vi "slider driver -- real.vi"(0 "slider in":refnum<vi>, 1 "slider action":T1, 9 "slider from":refnum<vi>, 11 "value IN":dbl=5700.934579439253, 12 "default":dbl=5700.934579439253) -> (4 "slider out":refnum<vi>, 6 "max":dbl, 8 "rel OUT":dbl, 10 "min":dbl, 15 "value OUT":dbl=5700.934579439253)   [LabVIEW 2018]
uses:
  slider action.ctl
  Q - not nan -- real.vi
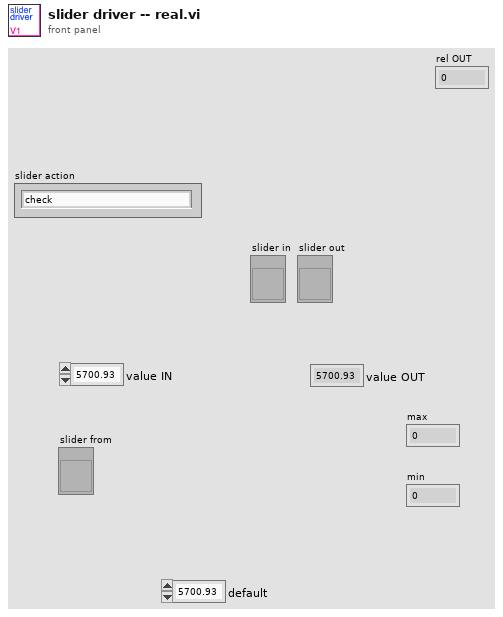
[diagram p1: front panel]
types:
  T1 = typedef "slider action.ctl" = enum16{"check", "copy range", "set from value", "set from ratio", "set from slider", "read using other slider", "set lower limit", "set upper limit", "set lower from slider", "set upper from slider"}
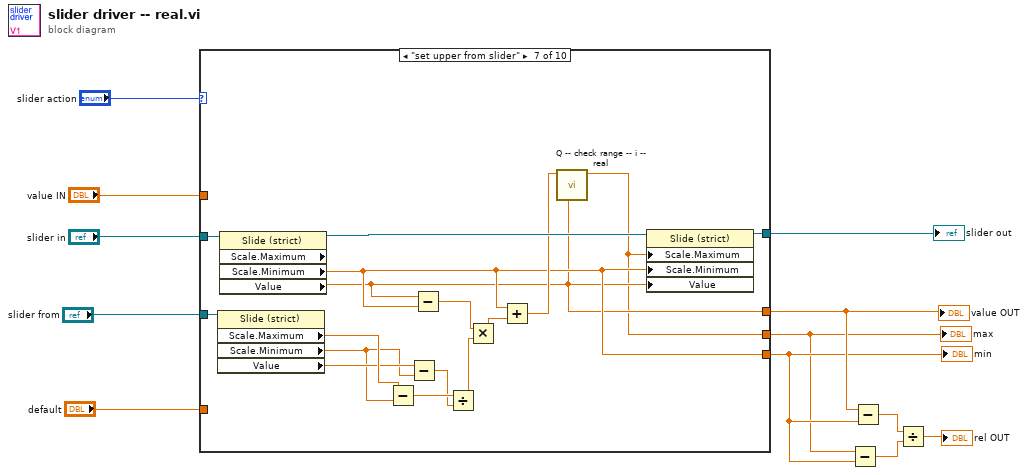
[diagram p0: block diagram]
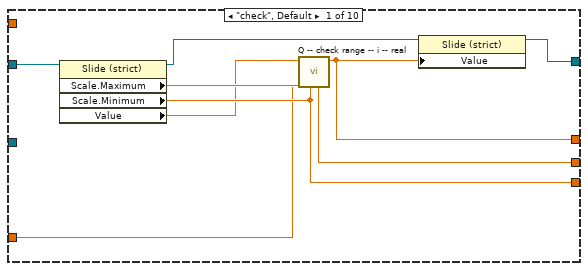
[diagram p2: hidden frame]
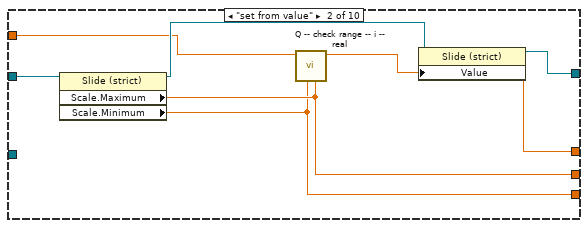
[diagram p3: hidden frame]
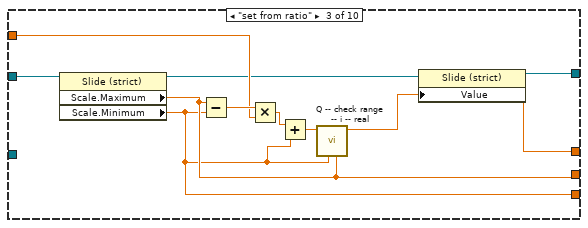
[diagram p4: hidden frame]
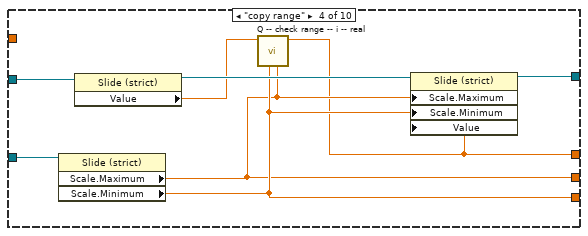
[diagram p5: hidden frame]
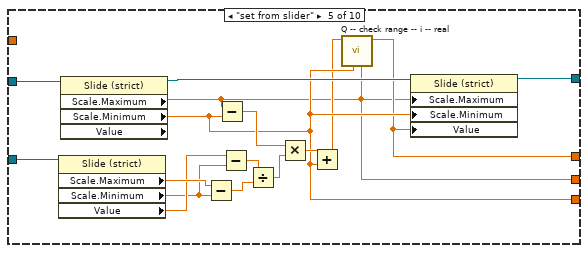
[diagram p6: hidden frame]
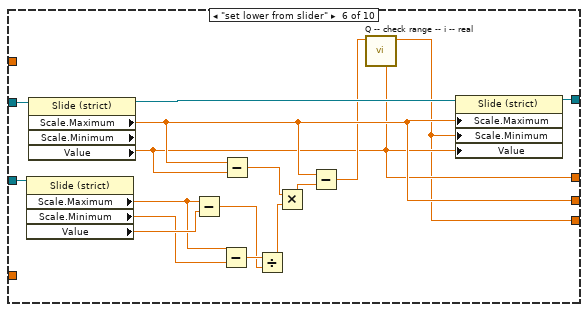
[diagram p7: hidden frame]
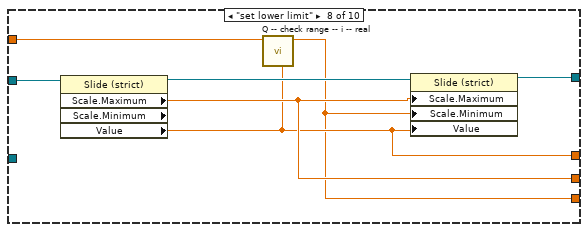
[diagram p8: hidden frame]
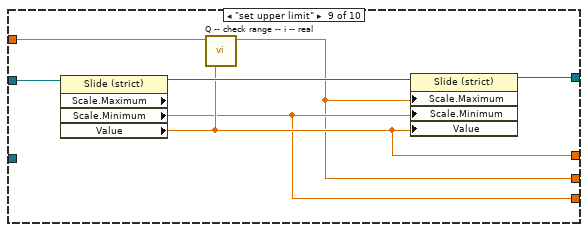
[diagram p9: hidden frame]
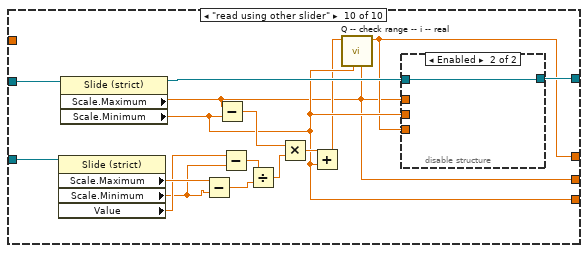
[diagram p10: hidden frame]
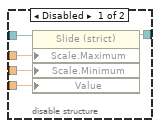
[diagram p11: hidden frame]
diagram:
  n1 = case shown="\"set upper from slider\"" "slider action" {
    tunnel: "slider in" -> [w20 w27 w37 w43 w59 w75 w91 w99 w106 w121]
    tunnel: [w19 w26 w36 w38 w47 w63 w79 w95 w103 w109] -> w6
    tunnel: [w17 w24 w35 w44 w60 w76 w92 w100 w107 w122] -> w2
    tunnel: "slider from" -> [_ _ _ w45 w61 w77 w93 _ _ w123]
    tunnel: [w15 w22 w30 w40 w49 w62 w80 w94 w102 w111] -> w5
    tunnel: [w16 w23 w34 w39 w46 w66 w78 w97 w101 w108] -> w4
    tunnel: "value IN" -> [_ w21 w32 _ _ _ _ w98 w105 _]
    tunnel: "default" -> [w14 _ _ _ _ _ _ _ _ _]
    frame "check", Default {
      n2 = property class="Slide (strict)"(reference=w20) -> (reference out=w18:refnum<vi>, "Scale.Maximum"=w16:dbl, "Scale.Minimum"=w15:dbl, "Value"=w13:dbl)  [unwired: 1 in, 1 out]
      n3 = call "Q -- check range -- i -- real.vi"("upper"=w16, "lower"=w15, "default"=w14, "number"=w13) -> ("number in range"=w19:dbl)  [unwired: 5 in, 2 out]
      n4 = property class="Slide (strict)"(reference=w18, "Value"=w19) -> (reference out=w17:refnum<vi>)  [unwired: 1 in, 1 out]
    }
    frame "set from value" {
      n5 = property class="Slide (strict)"(reference=w27) -> (reference out=w25:refnum<vi>, "Scale.Maximum"=w23:dbl, "Scale.Minimum"=w22:dbl)  [unwired: 1 in, 1 out]
      n6 = call "Q -- check range -- i -- real.vi"("upper"=w23, "lower"=w22, "number"=w21) -> ("number in range"=w26:dbl)  [unwired: 6 in, 2 out]
      n7 = property class="Slide (strict)"(reference=w25, "Value"=w26) -> (reference out=w24:refnum<vi>)  [unwired: 1 in, 1 out]
    }
    frame "set from ratio" {
      n8 = property class="Slide (strict)"(reference=w37) -> (reference out=w31:refnum<vi>, "Scale.Maximum"=w34:dbl, "Scale.Minimum"=w30:dbl)  [unwired: 1 in, 1 out]
      n9 = Subtract(x=w34, y=w30) -> (x-y=w33:dbl)
      n10 = Multiply(x=w33, y=w32) -> (x*y=w29:dbl)
      n11 = Add(x=w29, y=w30) -> (x+y=w28:dbl)
      n12 = call "Q -- check range -- i -- real.vi"("upper"=w34, "lower"=w30, "number"=w28) -> ("number in range"=w36:dbl)  [unwired: 6 in, 2 out]
      n13 = property class="Slide (strict)"(reference=w31, "Value"=w36) -> (reference out=w35:refnum<vi>)  [unwired: 1 in, 1 out]
    }
    frame "copy range" {
      n14 = property class="Slide (strict)"(reference=w45) -> ("Scale.Maximum"=w39:dbl, "Scale.Minimum"=w40:dbl)  [unwired: 1 in, 2 out]
      n15 = property class="Slide (strict)"(reference=w43) -> (reference out=w42:refnum<vi>, "Value"=w41:dbl)  [unwired: 1 in, 1 out]
      n16 = call "Q -- check range -- i -- real.vi"("upper"=w39, "lower"=w40, "number"=w41) -> ("number in range"=w38:dbl)  [unwired: 6 in, 2 out]
      n17 = property class="Slide (strict)"(reference=w42, "Scale.Maximum"=w39, "Scale.Minimum"=w40, "Value"=w38) -> (reference out=w44:refnum<vi>)  [unwired: 1 in, 1 out]
    }
    frame "set from slider" {
      n18 = property class="Slide (strict)"(reference=w61) -> ("Scale.Maximum"=w57:dbl, "Scale.Minimum"=w55:dbl, "Value"=w56:dbl)  [unwired: 1 in, 2 out]
      n19 = property class="Slide (strict)" props=["Scale", "Maximum", "Scale", "Minimum", "Value"](reference=w59) -> (reference out=w58:refnum<vi>, "Scale.Maximum"=w46:dbl, "Scale.Minimum"=w49:dbl)  [unwired: 1 in, 2 out]
      n20 = Subtract(x=w57, y=w55) -> (x-y=w53:dbl)
      n21 = Subtract(x=w46, y=w49) -> (x-y=w51:dbl)
      n22 = Subtract(x=w56, y=w55) -> (x-y=w54:dbl)
      n23 = Divide(x=w54, y=w53) -> (x/y=w52:dbl)
      n24 = Multiply(x=w51, y=w52) -> (x*y=w50:dbl)
      n25 = Add(x=w50, y=w49) -> (x+y=w48:dbl)
      n26 = call "Q -- check range -- i -- real.vi"("upper"=w46, "lower"=w49, "number"=w48) -> ("number in range"=w47:dbl)  [unwired: 6 in, 2 out]
      n27 = property class="Slide (strict)"(reference=w58, "Scale.Maximum"=w46, "Scale.Minimum"=w49, "Value"=w47) -> (reference out=w60:refnum<vi>)  [unwired: 1 in, 1 out]
    }
    frame "set lower from slider" {
      n28 = property class="Slide (strict)"(reference=w77) -> ("Scale.Maximum"=w71:dbl, "Scale.Minimum"=w70:dbl, "Value"=w72:dbl)  [unwired: 1 in, 2 out]
      n29 = property class="Slide (strict)" props=["Scale", "Maximum", "Scale", "Minimum", "Value"](reference=w75) -> (reference out=w74:refnum<vi>, "Scale.Maximum"=w66:dbl, "Value"=w63:dbl)  [unwired: 1 in, 2 out]
      n30 = Subtract(x=w71, y=w72) -> (x-y=w69:dbl)
      n31 = Subtract(x=w71, y=w70) -> (x-y=w73:dbl)
      n32 = Subtract(x=w66, y=w63) -> (x-y=w68:dbl)
      n33 = Divide(x=w73, y=w69) -> (x/y=w67:dbl)
      n34 = Multiply(x=w68, y=w67) -> (x*y=w65:dbl)
      n35 = Subtract(x=w66, y=w65) -> (x-y=w64:dbl)
      n36 = call "Q -- check range -- i -- real.vi"("upper"=w63, "number"=w64) -> ("number in range"=w62:dbl)  [unwired: 7 in, 2 out]
      n37 = property class="Slide (strict)"(reference=w74, "Scale.Maximum"=w66, "Scale.Minimum"=w62, "Value"=w63) -> (reference out=w76:refnum<vi>)  [unwired: 1 in, 1 out]
    }
    frame "set upper from slider" {
      n38 = property class="Slide (strict)"(reference=w93) -> ("Scale.Maximum"=w88:dbl, "Scale.Minimum"=w81:dbl, "Value"=w82:dbl)  [unwired: 1 in, 2 out]
      n39 = property class="Slide (strict)" props=["Scale", "Maximum", "Scale", "Minimum", "Value"](reference=w91) -> (reference out=w90:refnum<vi>, "Scale.Minimum"=w80:dbl, "Value"=w79:dbl)  [unwired: 1 in, 2 out]
      n40 = Subtract(x=w88, y=w81) -> (x-y=w89:dbl)
      n41 = Subtract(x=w82, y=w81) -> (x-y=w87:dbl)
      n42 = Subtract(x=w79, y=w80) -> (x-y=w86:dbl)
      n43 = Divide(x=w89, y=w87) -> (x/y=w85:dbl)
      n44 = Multiply(x=w86, y=w85) -> (x*y=w84:dbl)
      n45 = Add(x=w80, y=w84) -> (x+y=w83:dbl)
      n46 = call "Q -- check range -- i -- real.vi"("lower"=w79, "number"=w83) -> ("number in range"=w78:dbl)  [unwired: 7 in, 2 out]
      n47 = property class="Slide (strict)"(reference=w90, "Scale.Maximum"=w78, "Scale.Minimum"=w80, "Value"=w79) -> (reference out=w92:refnum<vi>)  [unwired: 1 in, 1 out]
    }
    frame "set lower limit" {
      n48 = property class="Slide (strict)" props=["Scale", "Maximum", "Scale", "Minimum", "Value"](reference=w99) -> (reference out=w96:refnum<vi>, "Scale.Maximum"=w97:dbl, "Value"=w95:dbl)  [unwired: 1 in, 2 out]
      n49 = call "Q -- check range -- i -- real.vi"("upper"=w95, "number"=w98) -> ("number in range"=w94:dbl)  [unwired: 7 in, 2 out]
      n50 = property class="Slide (strict)"(reference=w96, "Scale.Maximum"=w97, "Scale.Minimum"=w94, "Value"=w95) -> (reference out=w100:refnum<vi>)  [unwired: 1 in, 1 out]
    }
    frame "set upper limit" {
      n51 = property class="Slide (strict)" props=["Scale", "Maximum", "Scale", "Minimum", "Value"](reference=w106) -> (reference out=w104:refnum<vi>, "Scale.Minimum"=w102:dbl, "Value"=w103:dbl)  [unwired: 1 in, 2 out]
      n52 = call "Q -- check range -- i -- real.vi"("lower"=w103, "number"=w105) -> ("number in range"=w101:dbl)  [unwired: 7 in, 2 out]
      n53 = property class="Slide (strict)"(reference=w104, "Scale.Maximum"=w101, "Scale.Minimum"=w102, "Value"=w103) -> (reference out=w107:refnum<vi>)  [unwired: 1 in, 1 out]
    }
    frame "read using other slider" {
      n54 = property class="Slide (strict)"(reference=w123) -> ("Scale.Maximum"=w119:dbl, "Scale.Minimum"=w117:dbl, "Value"=w118:dbl)  [unwired: 1 in, 2 out]
      n55 = property class="Slide (strict)"(reference=w121) -> (reference out=w120:refnum<vi>, "Scale.Maximum"=w108:dbl, "Scale.Minimum"=w111:dbl)  [unwired: 1 in, 1 out]
      n56 = Subtract(x=w119, y=w117) -> (x-y=w115:dbl)
      n57 = Subtract(x=w108, y=w111) -> (x-y=w113:dbl)
      n58 = Subtract(x=w118, y=w117) -> (x-y=w116:dbl)
      n59 = Divide(x=w116, y=w115) -> (x/y=w114:dbl)
      n60 = Multiply(x=w113, y=w114) -> (x*y=w112:dbl)
      n61 = Add(x=w112, y=w111) -> (x+y=w110:dbl)
      n62 = call "Q -- check range -- i -- real.vi"("upper"=w108, "lower"=w111, "number"=w110) -> ("number in range"=w109:dbl)  [unwired: 6 in, 2 out]
      n63 = disable-structure shown="Enabled" {
        disable-tunnel: [w128 w129] -> w122
        disable-tunnel: w120 -> [w127 w129]
        disable-tunnel: w111 -> [w126 _]
        disable-tunnel: w109 -> [w125 _]
        disable-tunnel: w108 -> [w124 _]
        frame Disabled {
          n64 = property class="Slide (strict)"(reference=w127, "Scale.Maximum"=w124, "Scale.Minimum"=w126, "Value"=w125) -> (reference out=w128:refnum<vi>)  [unwired: 1 in, 1 out]
        }
        frame Enabled {
        }
      }
    }
  }
  "value OUT" <- w6
  "min" <- w5
  "max" <- w4
  "slider out" <- w2
  n65 = Subtract(x=w4, y=w5) -> (x-y=w7:dbl)
  n66 = Subtract(x=w6, y=w5) -> (x-y=w8:dbl)
  n67 = Divide(x=w8, y=w7) -> (x/y=→"rel OUT":dbl)
